vi "Ocean Server Parse Sentence.vi"(8 "error in (no error)":errorcluster, 11 "Ocean Server Sentence":string) -> (0 "error out":errorcluster, 3 "Values":T1)   [LabVIEW 2015, in "Compass Instrument.lvlib" / "Compass Instrument.lvclass"]
doc: "Parses the sentence and outputs the data."
uses:
  RDS Instruments/Compass Instrument/Compass Instrument.lvclass
  RDS Instruments/Compass/Compass Data.ctl
  RDS Instruments/RDS Instrument Library.lvlib
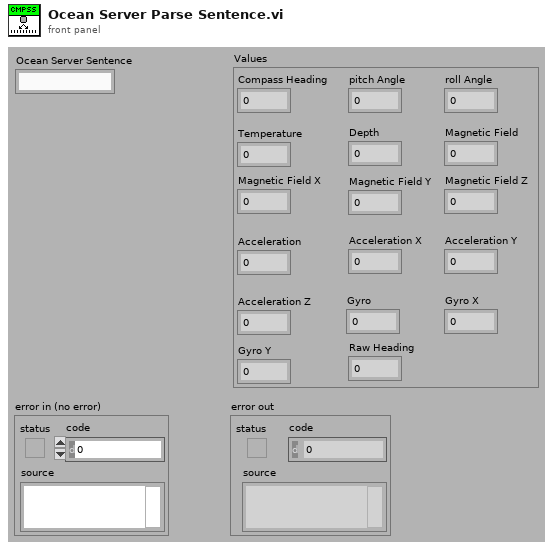
[diagram p1: front panel]
types:
  T1 = typedef "RDS Instrument Library.lvlib/Compass Data.ctl" = cluster{"Compass Heading":sgl, "pitch Angle":sgl, "roll Angle":sgl, "Temperature":sgl, "Depth":sgl, "Magnetic Field":sgl, "Magnetic Field X":sgl, "Magnetic Field Y":sgl, "Magnetic Field Z":sgl, "Acceleration":sgl, "Acceleration X":sgl, "Acceleration Y":sgl, "Gyro":sgl, "Gyro X":sgl, "Acceleration Z":sgl, "Gyro Y":sgl, "Raw Heading":sgl}
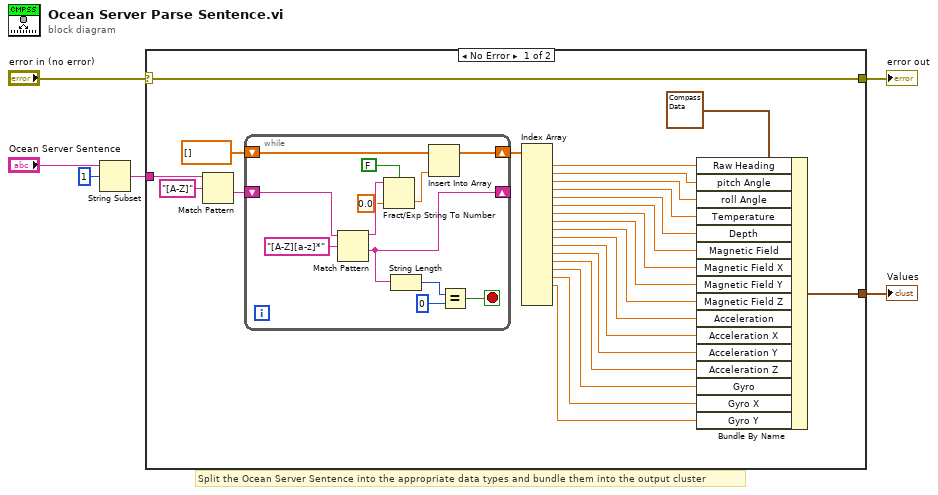
[diagram p0: block diagram]
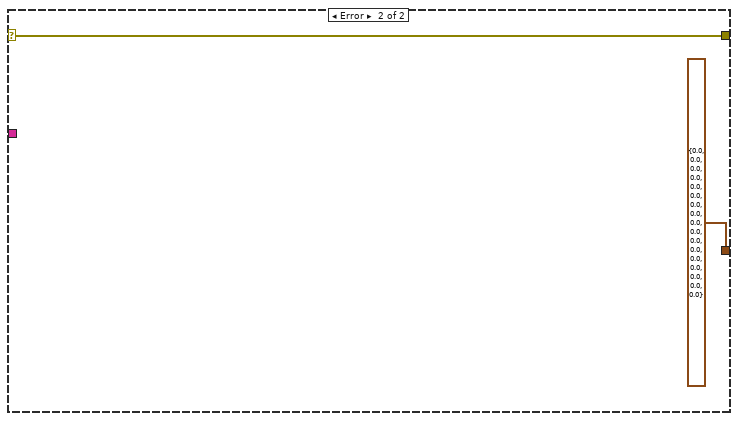
[diagram p2: hidden frame]
diagram:
  # "Split the Ocean Server Sentence into the appropriate data types and bundle them into the output cluster"
  n1 = String Subset(string="Ocean Server Sentence", offset (0)=1) -> (substring=w4:string)  [unwired: 1 in]
  n2 = case shown="No Error" "error in (no error)" {
    selector: "error in (no error)" -> [w9 w44]
    tunnel: w4 -> [w28 _]
    tunnel: [w9 w44] -> w5
    tunnel: [w8 T1 {"Compass Heading"=0.0, "pitch Angle"=0.0, "roll Angle"=0.0, "Temperature"=0.0, "Depth"=0.0, "Magnetic Field"=0.0, "Magnetic Field X"=0.0, "Magnetic Field Y"=0.0, "Magnetic Field Z"=0.0, "Acceleration"=0.0, "Acceleration X"=0.0, "Acceleration Y"=0.0, "Gyro"=0.0, "Gyro X"=0.0, "Acceleration Z"=0.0, "Gyro Y"=0.0, "Raw Heading"=0.0} ("Values")] -> w1
    frame No Error {
      n3 = Match Pattern(string=w28, regular expression="[A-Z]") -> (after substring=w27:string)  [unwired: 1 in, 3 out]
      n4 = while {
        shift-right: [w38] -> w26
        shift-left: sgl[] [] ("array") -> [w39]
        shift-right: [w37] -> _
        shift-left: w27 -> [w33]
        stop <- w34 stop-if-true
        n5 = Match Pattern(string=w33, regular expression="[A-Z][a-z]*") -> (before substring=w41:string, after substring=w37:string)  [unwired: 1 in, 2 out]
        n6 = Fract/Exp String To Number(use system decimal point (T)=FALSE, string=w41, default (0 dbl)=sgl 0.0 ("default (0 DBL)")) -> (number=w40:sgl)  [unwired: 1 in, 1 out]
        n7 = String Length(string=w37) -> (length=w36:i32)
        n8 = Insert Into Array(array=w39, new element=w40) -> (w38:sgl[])  [unwired: 1 in]
        n9 = Equal?(x=w36, y=0) -> (x = y?=w34:bool)
      }
      n10 = Index Array(array=w26) -> (element #1=w25:sgl, element #2=w24:sgl, element #3=w23:sgl, element #4=w22:sgl, element #5=w21:sgl, element #6=w20:sgl, element #7=w19:sgl, element #8=w18:sgl, element #9=w17:sgl, element #10=w16:sgl, element #11=w15:sgl, element #12=w14:sgl, element #13=w13:sgl, element #14=w12:sgl, element #15=w11:sgl, element #16=w10:sgl)  [unwired: 18 in, 2 out]
      n11 = Bundle By Name(cluster=T1 {"Compass Heading"=0.0, "pitch Angle"=0.0, "roll Angle"=0.0, "Temperature"=0.0, "Depth"=0.0, "Magnetic Field"=0.0, "Magnetic Field X"=0.0, "Magnetic Field Y"=0.0, "Magnetic Field Z"=0.0, "Acceleration"=0.0, "Acceleration X"=0.0, "Acceleration Y"=0.0, "Gyro"=0.0, "Gyro X"=0.0, "Acceleration Z"=0.0, "Gyro Y"=0.0, "Raw Heading"=0.0} ("Values"), "Raw Heading"=w25, "pitch Angle"=w24, "roll Angle"=w23, "Temperature"=w22, "Depth"=w21, "Magnetic Field"=w20, "Magnetic Field X"=w19, "Magnetic Field Y"=w18, "Magnetic Field Z"=w17, "Acceleration"=w16, "Acceleration X"=w15, "Acceleration Y"=w14, "Acceleration Z"=w13, "Gyro"=w12, "Gyro X"=w11, "Gyro Y"=w10) -> (w8:T1)
    }
    frame Error {
    }
  }
  "error out" <- w5
  "Values" <- w1
